vi "3.1.vi"() -> ()   [LabVIEW 2017]
panel:
  out "?":dbl
  in  "x2":dbl
  out "y1":dbl
  in  "x1":dbl
  # "y2"
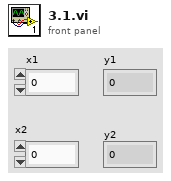
[diagram p1: front panel]
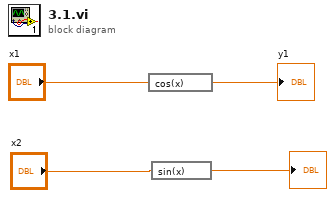
[diagram p0: block diagram]
diagram:
  n1 = expression code="cos(x)"("x1") -> (→"y1":dbl)
  n2 = expression code="sin(x)"("x2") -> (→"?":dbl)
